vi "IV.vi"(2 "Run uninterrupted?":bool, 3 "Device Category IN:":string(combo)="Short Strip" caption="Device Category:", 4 "Batch No. IN:":string caption="Batch No.:", 5 "Sensor Serial No. IN:":string caption="Sensor Serial No.:", 6 "DB Serial No. IN:":string caption="DB Serial No.:") -> (0 "Done!":bool)   [LabVIEW 2018]
doc: "Performs IV measurements according to ATLAS ITk Quality Control Specifications."
uses:
  general_VIs/globals/QC_MeasurementSetup.vi
  general_VIs/globals/QC_RunInformation.vi
  InstrControl/InstrumentSetup.vi
  InstrControl/Switching/Switching.lvclass
  InstrControl/SupplyControl/SupplyControl.lvclass
  InstrControl/ArduinoControl/ArduinoControl.lvclass
  <vilib>/Analysis/NI_AALBase.lvlib
  InstrControl/InstrControl.lvclass
panel:
  out "Tab Control 2":enum32{"IV Setup", "IV Scan"}(tab)
  in  "V_breakdown limit [V]":dbl=-500.0
  in  "Set current limit?":bool
  in  "Current Limit [µA]":dbl=1000.0 min=0.0001 format="%.3f"
  in  "Measurement Configurations":bool
  in  "hold steps IN":i32=6 caption="hold steps"
  in  "Initial volts [V] IN":dbl caption="Initial volts [V]"
  in  "Final volts [V] IN":dbl=-700.0 caption="Final volts [V]"
  in  "step [V] IN":dbl=10.0 caption="step [V]" format="%.1f"
  in  "step interval [s] IN":i32=10 caption="step interval [s]"
  in  "Continue":bool
  in  "Quit":bool
  out "hold steps":i32
  out "RH":dbl[](array[numeric]) caption="RH [%]" format="%#.2f"
  out "Temp.":dbl[](array[numeric]) caption="Temp. [°C]" format="%#.2f"
  out "Current":dbl[](array[numeric]) caption="Current [nA]"
  out "Volts":dbl[](array[numeric]) caption="Volts [V]"
  out "step interval [s]":i32=10
  out "step [V]":dbl=10.0 format="%.1f"
  out "Final volts [V]":dbl=-700.0 format="%.1f"
  out "Initial volts [V]":dbl format="%.1f"
  out "Igraph":cluster{dbl[], dbl[]}(graph)
  in  "Scales":T1(ring)
  in  "Iscale":enum16{"nanoAmps", "microAmps", "milliAmps"}(ring)
  out "positive ramp?":bool
  out "Tab Control":enum32{"IV Setup", "IV Scan"}(tab)
  in  "Hardware Configurations":bool
  in  "User:":string(combo)="Christoph"
  in  "IV Supply":string(combo)="Keithley 2410"
  in  "Temperature":enum16{"Read Arduino", "Enter manually"}(ring)
  in  "Manufacturer:":string(combo)="Hamamatsu"
  in  "abort":bool
  out "Device Category:":string
  out "DB Serial No.:":string
  out "Current Volts:":dbl format="%.2f"
  in  "quit (no save)":bool
  in  "Quit & Save":bool
  out "Bias On/Off:":bool
  out "STATUS 1":string
  out "Initiated:":string
  out "Sensor No.:":string
  out "No of steps":u32
  out "Current reading No.":u32
  out "Last reading at:":string
  # "University of\nCambridge"
  # "Strip Sensor QC: IV"
  # "Vertical Scale:"
  # "Measurement Configuration"
  # "IV Scan parameters:"
  # "Last 5 readings:"
  # "n-4"
  # "n-3"
  # "n-2"
  # "n-1"
  # "n"
  # "DUT Description"
  # "Hardware"
  # "DUT & Test Description:"
  # "Current status:"
  # "Rdg No:"
  # "out of"
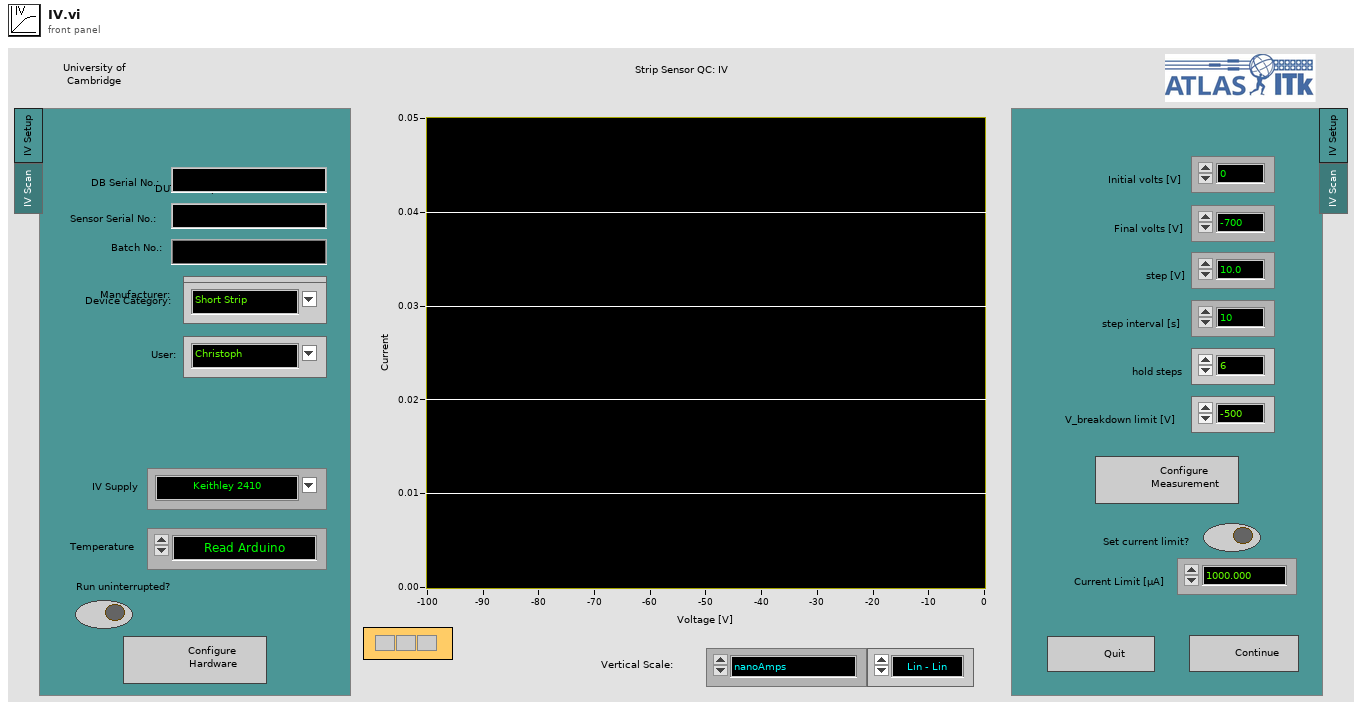
[diagram p1: front panel]
types:
  T1 = enum16{"Lin - Lin", "Log - Lin", "Lin - Log", "Log - log"}
  T2 = enum16{"Supply", "LCR", "Multimeter", "Switching"}
  T3 = enum16{"Reset", "Read Array", "Read Element", "Write Element", "Write Array", "Add Element", "Add Array"}
  T4 = enum16{"Reset", "Ground", "Striptest SMU", "Striptest LCR", "IV", "CV", "Interstrip Cap", "Interstrip Res"}
  T5 = enum32{"IV", "CV", "Stability", "Striptest", "Cis", "Ris", "PTP"}
  T6 = cluster{"Sensor Serial No.:":string, "Wafer Serial No.:":string, "Batch:":string, "Manufacturer:":string, "Device Category:":string, "Database Serial No.:":string, "Date Initiated:":string, "Time Initiated:":string, "Test":string, "Instruments used:":string, "Probeplan used:":string, "End of Run comment:":string, "User:":string}
  T7 = cluster{"Institute":string, "Manufacturers":string[], "Devices":string[], "Serialnumbers Lookup DB":string, "Data directory":string, "Backup & screenshot directory":string, "List of known users":string[]}
  T8 = cluster{"Supply":refnum<class "SupplyControl.lvclass">, "Initial Voltage [V]":dbl, "Final Voltage [V]":dbl, "Step Size [V]":dbl, "Step Interval [s]":i32, "Number Of Steps":u32, "Ramp down steps [V]":dbl, "Ramp down Interval [s]":i32, "hold steps":i32, "Set Current Limit?":bool, "Current Limit [µA]":dbl, "Temperature Readout":enum16{"Read Arduino", "Enter manually"}, "Arduino":refnum<class "ArduinoControl.lvclass">, "Supply Name":string, "V_breakdown Limit [V]":dbl, "Switching":refnum<class "Switching.lvclass">, "Matrix used?":bool, "Matrix X Channels":cluster{"Bias Supply / SMU LO":i32, "Bias Supply / SMU HI":i32, "CV Box LO":i32, "CV Box HI":i32, "CV Box LO IN":i32, "CV Box HI IN":i32, "Volt meter LO":i32, "Volt meter HI":i32, "Mux1 C1":i32, "Mux1 C2":i32, "Mux2 C1":i32, "Mux2 C2":i32}, "IV Test?":bool}
  T9 = cluster{"VISA address":refnum<visa-resource-name>, "T sensor":enum16{"SHT", "DS"}, "Arduino":refnum<class "ArduinoControl.lvclass">}
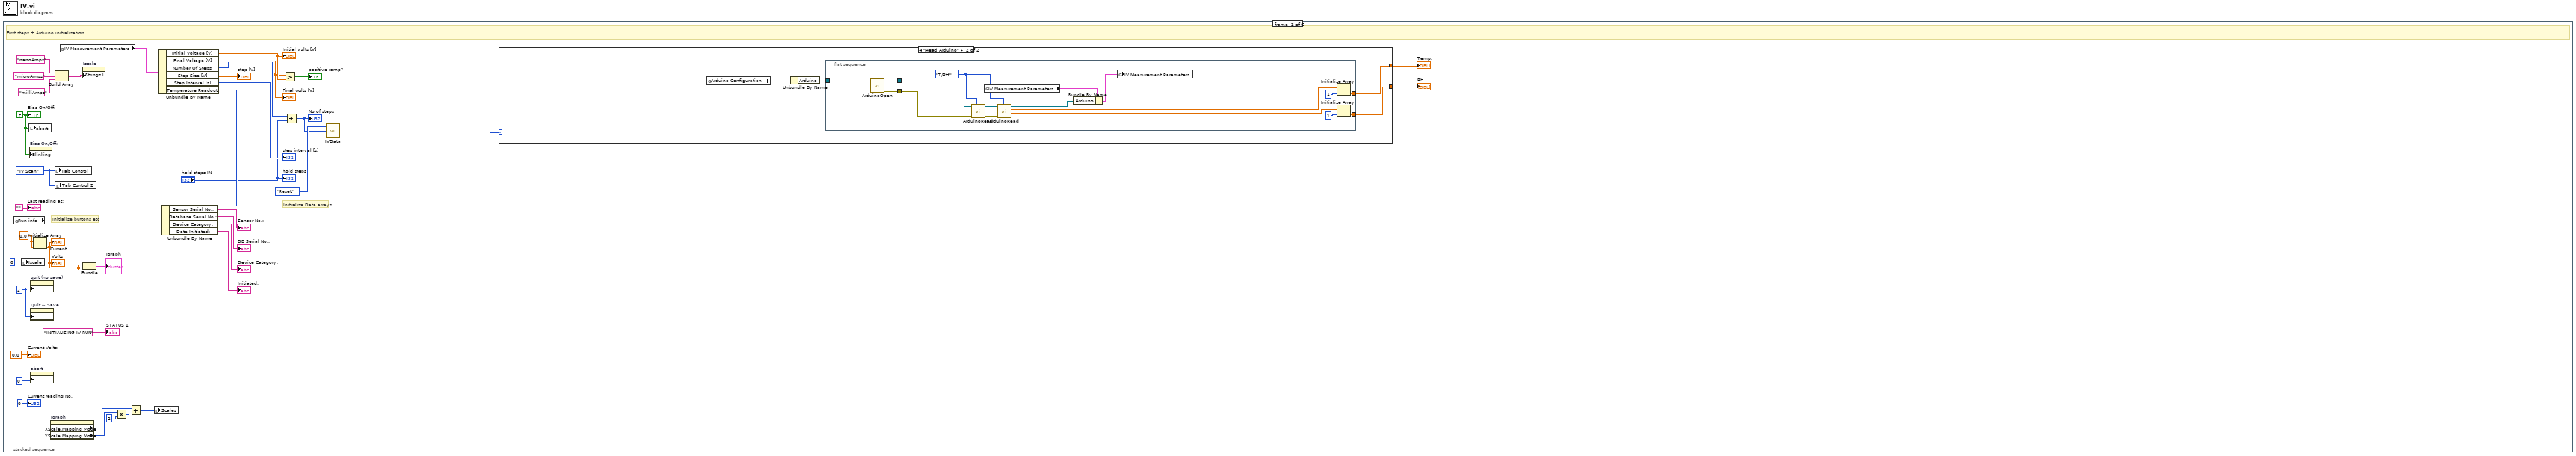
[diagram p0: block diagram]
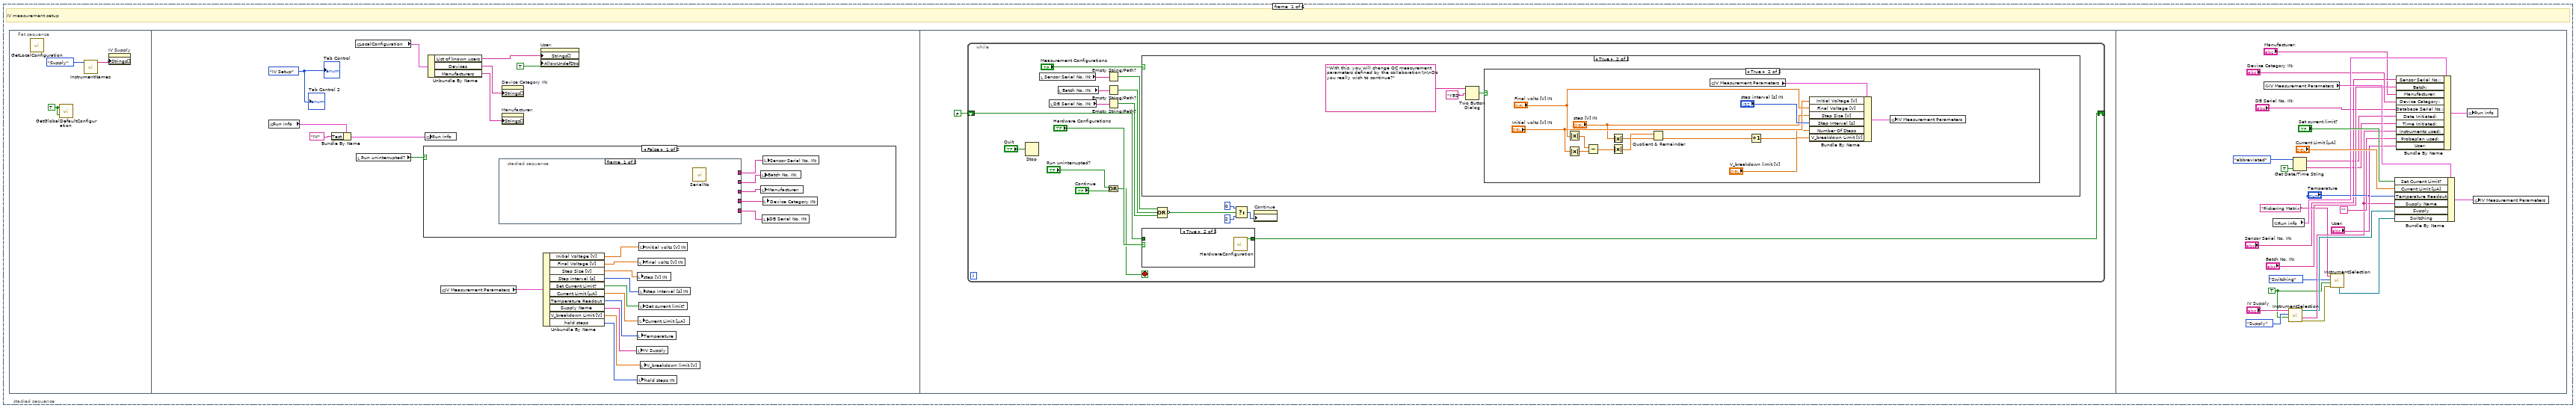
[diagram p2: hidden frame]
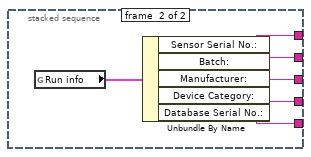
[diagram p3: hidden frame]
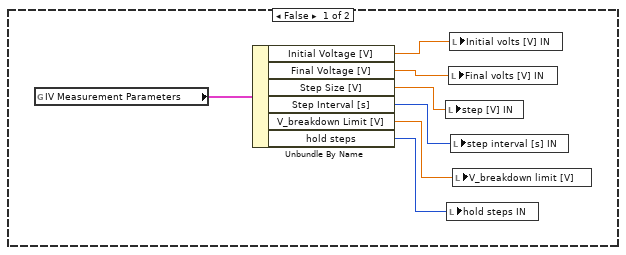
[diagram p6: hidden frame]
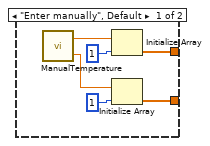
[diagram p8: hidden frame]
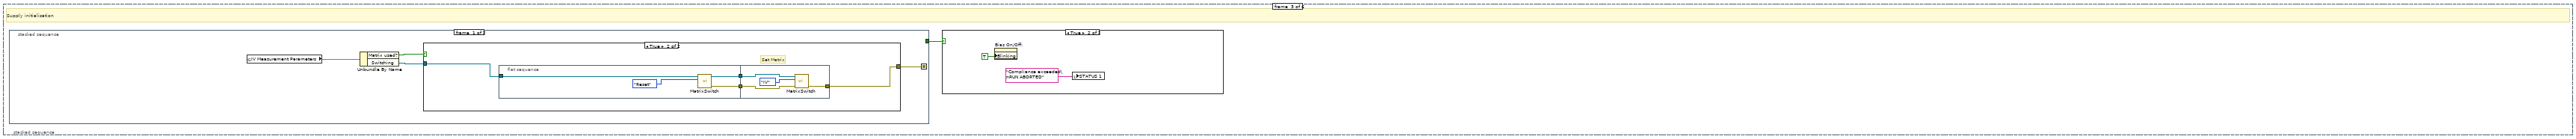
[diagram p9: hidden frame]
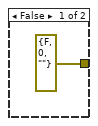
[diagram p10: hidden frame]
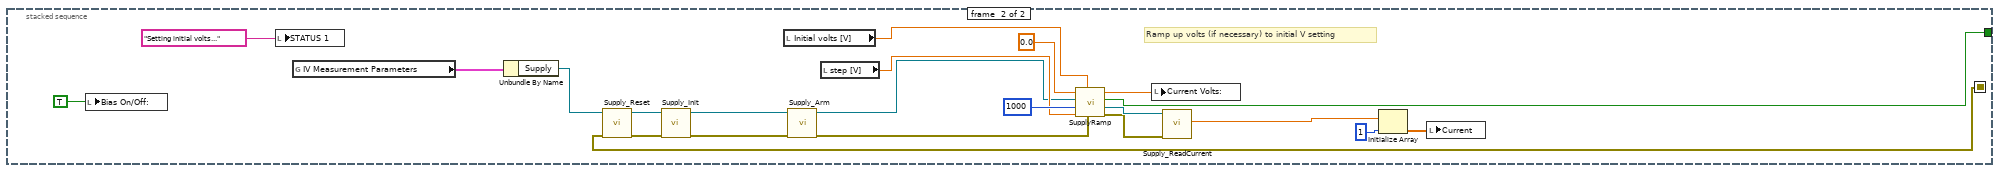
[diagram p11: hidden frame]
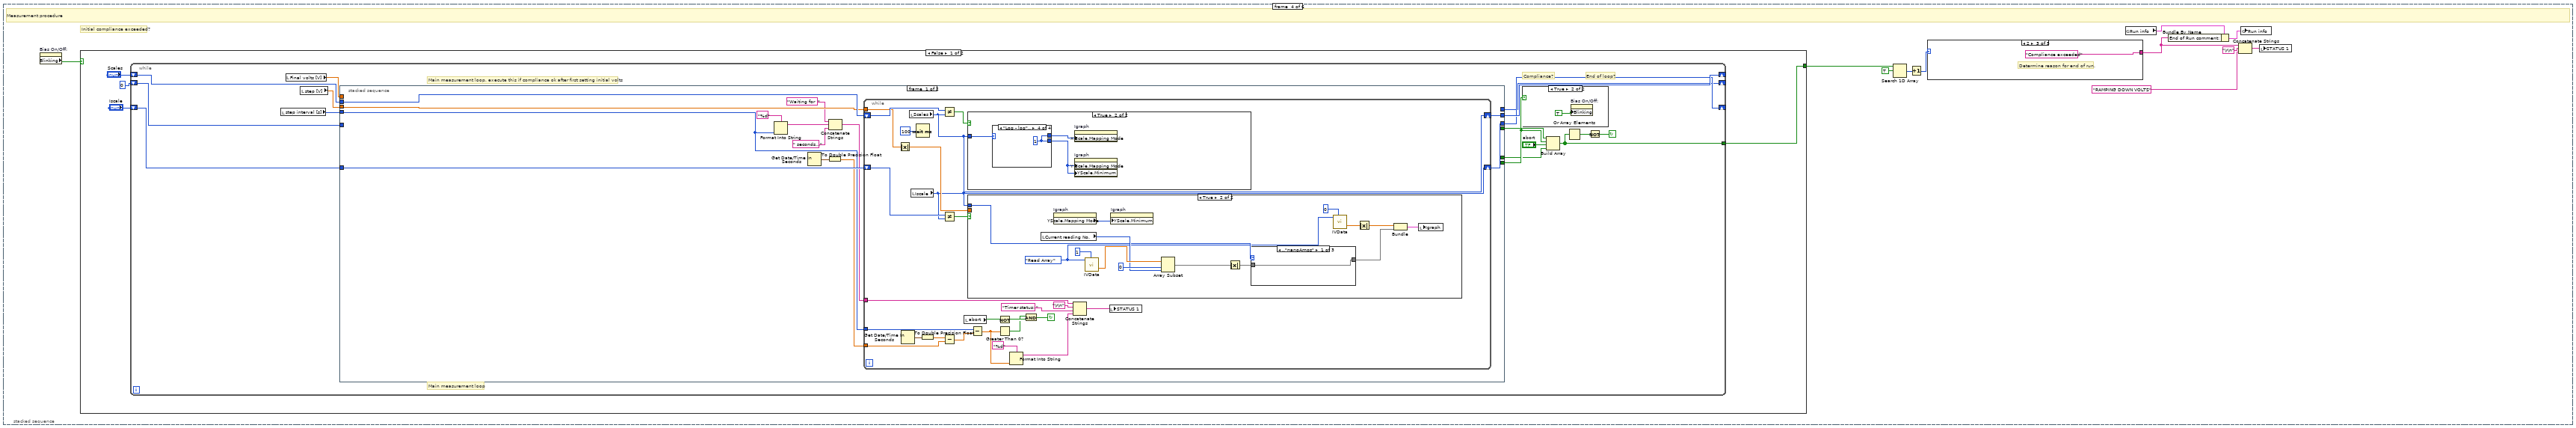
[diagram p13: hidden frame]
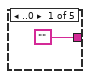
[diagram p14: hidden frame]
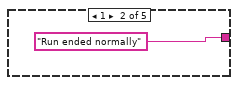
[diagram p15: hidden frame]
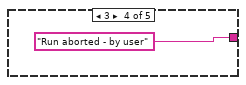
[diagram p16: hidden frame]
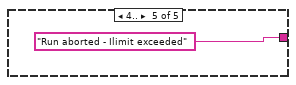
[diagram p17: hidden frame]
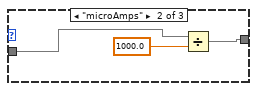
[diagram p19: hidden frame]
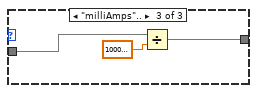
[diagram p20: hidden frame]
diagram:
  n1 = stacked-sequence {
    frame #0 {
      # "IV measurement setup"
      n2 = flat-sequence {
        frame #0 {
          w3 = TRUE
          n3 = call "GetLocalConfiguration.vi"() -> ()  [unwired: 3 in, 1 out]
          n4 = call "GetGlobalDefaultConfiguration.vi"("DO NOT override instruments"=w3, "Read defaults?"=w3) -> ()  [unwired: 1 in, 1 out]
          n5 = call "InstrumentNames.vi"("Instrument type"=T2."Supply") -> ("Instrument names"=w1:string[])  [unwired: 9 in, 1 out]
          n6 = property on="IV Supply" class="CmbBox"("Strings[]"=w1) -> ()  [unwired: 2 in, 2 out]
        }
        frame #1 {
          w12 = enum32{"IV Setup", "IV Scan"}."IV Setup" ("Tab Control")
          n7 = global read "QC_RunInformation.vi" "Run info"() -> (w15:T6)
          n8 = Bundle By Name(cluster=w15, "Test"="IV") -> (w13:T6)
          n9 = global read "QC_RunInformation.vi" "LocalConfiguration"() -> (w19:T7)
          n10 = local read "Run uninterrupted?"() -> (w16:bool)
          n11 = case shown="False" w16 {
            frame False {
              n12 = stacked-sequence {
                tunnel: [_ w35] -> w28
                tunnel: [_ w34] -> w27
                tunnel: [_ w33] -> w26
                tunnel: [_ w32] -> w29
                tunnel: [_ w30] -> w25
                frame #0 {
                  n13 = call "SerialNo.vi"() -> ()  [unwired: 5 in, 1 out]
                }
                frame #1 {
                  n14 = global read "QC_RunInformation.vi" "Run info"() -> (w31:T6)
                  n15 = Unbundle By Name(w31) -> ("Sensor Serial No.:"=w35:string, "Batch:"=w34:string, "Manufacturer:"=w33:string, "Device Category:"=w32:string, "Database Serial No.:"=w30:string)
                }
              }
              n16 = local write "Batch No. IN:"(w27) -> ()
              n17 = local write "Manufacturer:"(w26) -> ()
              n18 = local write "DB Serial No. IN:"(w25) -> ()
              n19 = local write "Device Category IN:"(w29) -> ()
              n20 = local write "Sensor Serial No. IN:"(w28) -> ()
            }
            frame True {
            }
          }
          n21 = global write "QC_RunInformation.vi" "Run info"(w13) -> ()
          n22 = Unbundle By Name(w19) -> ("List of known users"=w18:string[], "Devices"=w5:string[], "Manufacturers"=w4:string[])
          n23 = global read "QC_MeasurementSetup.vi" "IV Measurement Parameters"() -> (w22:T8)
          n24 = property on="Device Category IN:" class="CmbBox"("Strings[]"=w5) -> ()  [unwired: 2 in, 2 out]
          n25 = property on="Manufacturer:" class="CmbBox"("Strings[]"=w4) -> ()  [unwired: 2 in, 2 out]
          n26 = property on="User:" class="CmbBox"("Strings[]"=w18, "AllowUndefStrs"=TRUE) -> ()  [unwired: 2 in, 2 out]
          n27 = Unbundle By Name(w22) -> ("Initial Voltage [V]"=w10:dbl, "Final Voltage [V]"=w9:dbl, "Step Size [V]"=w8:dbl, "Step Interval [s]"=w11:i32, "Set Current Limit?"=w21:bool, "Current Limit [µA]"=w20:dbl, "Temperature Readout"=w24:enum16{"Read Arduino", "Enter manually"}, "Supply Name"=w23:string, "V_breakdown Limit [V]"=w7:dbl, "hold steps"=w6:i32)
          n28 = local write "IV Supply"(w23) -> ()
          n29 = local write "step [V] IN"(w8) -> ()
          n30 = local write "Temperature"(w24) -> ()
          n31 = local write "hold steps IN"(w6) -> ()
          n32 = local write "Final volts [V] IN"(w9) -> ()
          n33 = local write "Current Limit [µA]"(w20) -> ()
          n34 = local write "Initial volts [V] IN"(w10) -> ()
          n35 = local write "Set current limit?"(w21) -> ()
          n36 = local write "step interval [s] IN"(w11) -> ()
          n37 = local write "V_breakdown limit [V]"(w7) -> ()
          "Tab Control" <- w12
          "Tab Control 2" <- w12
        }
        frame #2 {
          n38 = while {
            shift-right: [w44] -> _
            shift-left: FALSE -> [w43]
            stop <- w40 stop-if-true
            n39 = Stop(stop? (T)="Quit") -> ()
            n40 = local read "Sensor Serial No. IN:"() -> (w53:string)
            n41 = local read "DB Serial No. IN:"() -> (w38:string)
            n42 = local read "Batch No. IN:"() -> (w46:string)
            n43 = Empty String/Path?(string/path=w53) -> (empty?=w52:bool)
            n44 = Empty String/Path?(string/path=w46) -> (empty?=w45:bool)
            n45 = Empty String/Path?(string/path=w38) -> (empty?=w37:bool)
            n46 = Or(x="Run uninterrupted?", y="Continue") -> (x .or. y?=w40:bool)
            n47 = case shown="True" "Measurement Configurations" {
              frame False {
              }
              frame True {
                n48 = Two Button Dialog(message="With this, you will change QC measurement parameters defined by the collaboration!\n\nDo you really wish to continue?", 2:"YES") -> (T button?=w55:bool)  [unwired: 1 in]
                n49 = case shown="True" w55 {
                  frame False {
                    n50 = global read "QC_MeasurementSetup.vi" "IV Measurement Parameters"() -> (w64:T8)
                    n51 = Unbundle By Name(w64) -> ("Initial Voltage [V]"=w62:dbl, "Final Voltage [V]"=w63:dbl, "Step Size [V]"=w61:dbl, "Step Interval [s]"=w60:i32, "V_breakdown Limit [V]"=w59:dbl, "hold steps"=w58:i32)
                    n52 = local write "step [V] IN"(w61) -> ()
                    n53 = local write "hold steps IN"(w58) -> ()
                    n54 = local write "Final volts [V] IN"(w63) -> ()
                    n55 = local write "Initial volts [V] IN"(w62) -> ()
                    n56 = local write "step interval [s] IN"(w60) -> ()
                    n57 = local write "V_breakdown limit [V]"(w59) -> ()
                  }
                  frame True {
                    n58 = Absolute Value(x="Final volts [V] IN") -> (abs(x)=w74:dbl)
                    n59 = Absolute Value(x="Initial volts [V] IN") -> (abs(x)=w73:dbl)
                    n60 = Subtract(x=w74, y=w73) -> (x-y=w68:dbl)
                    n61 = Absolute Value(x="step [V] IN") -> (abs(x)=w69:dbl)
                    n62 = Absolute Value(x=w68) -> (abs(x)=w70:dbl)
                    n63 = Quotient & Remainder(x=w70, y=w69) -> (floor(x/y)=w66:dbl)  [unwired: 1 out]
                    n64 = global read "QC_MeasurementSetup.vi" "IV Measurement Parameters"() -> (w78:T8)
                    n65 = Increment(x=w66) -> (x+1=w65:dbl)
                    n66 = Bundle By Name(cluster=w78, "Initial Voltage [V]"="Initial volts [V] IN", "Final Voltage [V]"="Final volts [V] IN", "Step Size [V]"="step [V] IN", "Step Interval [s]"="step interval [s] IN", "Number Of Steps"=w65, "V_breakdown Limit [V]"="V_breakdown limit [V]") -> (w75:T8)
                    n67 = global write "QC_MeasurementSetup.vi" "IV Measurement Parameters"(w75) -> ()
                  }
                }
              }
            }
            n68 = case shown="True" "Hardware Configurations" {
              tunnel: [w79 w80] -> w44
              tunnel: w43 -> [w79 _]
              frame False {
              }
              frame True {
                n69 = call "HardwareConfiguration.vi"() -> ("configured?"=w80:bool)  [unwired: 11 in]
              }
            }
            n70 = Compound Arithmetic op=OR(w52, w45, w37) -> (invert w51:bool)
            n71 = Select(t=0, s=w51, f=2) -> (s? t:f=w48:i32)
            n72 = property on="Continue" class="Bool"("DisabledEnum"=w48) -> ()  [unwired: 2 in, 2 out]
          }
        }
        frame #3 {
          w88 = TRUE
          n73 = global read "QC_MeasurementSetup.vi" "IV Measurement Parameters"() -> (w106:T8)
          n74 = global read "QC_RunInformation.vi" "Run info"() -> (w101:T6)
          n75 = call "InstrumentSelection.vi"("Verify GPIB address"=w88, "Instrument type"=T2."Supply", "Instrument name IN"="IV Supply") -> ("error out"=w90:errorcluster, "Instrument name OUT"=w93:string, "Supply"=w92:refnum<class "SupplyControl.lvclass">)  [unwired: 3 in, 3 out]
          n76 = Get Date/Time String(date format (0)=enum16{"short", "long", "abbreviated"}."abbreviated", want seconds? (F)=TRUE) -> (date string=w82:string, time string=w81:string)  [unwired: 1 in]
          n77 = call "InstrumentSelection.vi"("error in (no error)"=w90, "Verify GPIB address"=w88, "Instrument type"=T2."Switching", "Instrument name IN"="Pickering Matrix") -> ("Switching"=w89:refnum<class "Switching.lvclass">)  [unwired: 2 in, 5 out]
          n78 = Bundle By Name(cluster=w106, "Set Current Limit?"="Set current limit?", "Current Limit [µA]"="Current Limit [µA]", "Temperature Readout"="Temperature", "Supply Name"=w93, "Supply"=w92, "Switching"=w89) -> (w107:T8)
          n79 = Bundle By Name(cluster=w101, "Sensor Serial No.:"="Sensor Serial No. IN:", "Batch:"="Batch No. IN:", "Manufacturer:"="Manufacturer:", "Device Category:"="Device Category IN:", "Database Serial No.:"="DB Serial No. IN:", "Date Initiated:"=w82, "Time Initiated:"=w81, "Instruments used:"=w93, "Probeplan used:"="", "User:"="User:") -> (w100:T6)
          n80 = global write "QC_RunInformation.vi" "Run info"(w100) -> ()
          n81 = global write "QC_MeasurementSetup.vi" "IV Measurement Parameters"(w107) -> ()
        }
      }
    }
    frame #1 {
      w109 = enum32{"IV Setup", "IV Scan"}."IV Scan" ("Tab Control")
      w129 = 2
      w136 = 0.0
      w128 = FALSE ("Visible")
      # "Initialise buttons etc"
      # "Initialise Data arrays"
      # "First steps + Arduino initialisation"
      n82 = global read "QC_RunInformation.vi" "Run info"() -> (w145:T6)
      n83 = local write "Iscale"(u16 0 ("Scale")) -> ()
      n84 = local write "abort"(w128) -> ()
      n85 = property on="Bias On/Off:" class="Bool (strict)"("Blinking"=w128) -> ()  [unwired: 2 in, 2 out]
      n86 = property on="quit (no save)" class="Bool"("DisabledEnum"=w129) -> ()  [unwired: 2 in, 2 out]
      n87 = property on="Quit & Save" class="Bool"("DisabledEnum"=w129) -> ()  [unwired: 2 in, 2 out]
      n88 = property on="abort" class="Bool (strict)"("DisabledEnum"=0) -> ()  [unwired: 2 in, 2 out]
      n89 = Initialize Array(w136, w136) -> (w111:dbl[])
      "Volts" <- w111
      "Current" <- w111
      n90 = property on="Igraph" class="XYGraph (strict)"() -> ("XScale.Mapping Mode"=w121:u8, "YScale.Mapping Mode"=w120:u8)  [unwired: 2 in, 2 out]
      n91 = local write "Tab Control"(w109) -> ()
      n92 = Build Array("nanoAmps", "microAmps", "milliAmps") -> (w142:string[])
      n93 = local write "Tab Control 2"(w109) -> ()
      n94 = global read "QC_MeasurementSetup.vi" "IV Measurement Parameters"() -> (w117:T8)
      n95 = property on="Iscale" class="Enum (strict)"("Strings []"=w142) -> ()  [unwired: 2 in, 2 out]
      n96 = Bundle(w111, w111) -> (→"Igraph":cluster{dbl[], dbl[]})  [unwired: 1 in]
      n97 = Multiply(x=w120, y=2) -> (x*y=w123:i32)
      n98 = Add(x=w121, y=w123) -> (x+y=w119:i32)
      n99 = local write "Scales"(w119) -> ()
      n100 = Unbundle By Name(w117) -> ("Initial Voltage [V]"=w127:dbl, "Final Voltage [V]"=w126:dbl, "Number Of Steps"=w113:u32, "Step Size [V]"=→"step [V]":dbl, "Step Interval [s]"=→"step interval [s]":i32, "Temperature Readout"=w130:enum16{"Read Arduino", "Enter manually"})
      "Initial volts [V]" <- w127
      "Final volts [V]" <- w126
      n101 = Unbundle By Name(w145) -> ("Sensor Serial No.:"=→"Sensor No.:":string, "Database Serial No.:"=→"DB Serial No.:":string, "Device Category:"=→"Device Category:":string, "Date Initiated:"=→"Initiated:":string)
      n102 = Greater?(x=w126, y=w127) -> (0:→"positive ramp?":bool)
      n103 = Add(x=w113, y="hold steps IN") -> (x+y=w112:u32)
      "No of steps" <- w112
      n104 = call "IVData.vi"("Action"=T3."Reset", "Array Size / Index"=w112) -> ()  [unwired: 3 in, 2 out]
      n105 = case shown="\"Read Arduino\"" w130 {
        tunnel: [w151 w158] -> w133
        tunnel: [w148 w157] -> w118
        frame "Enter manually", Default {
          n106 = call "ManualTemperature.vi"() -> ("Humidity [%] out"=w147:dbl, "Temperature [°C] out"=w152:dbl)
          n107 = Initialize Array(w152, 1) -> (w151:dbl[])
          n108 = Initialize Array(w147, 1) -> (w148:dbl[])
        }
        frame "Read Arduino" {
          n109 = global read "InstrumentSetup.vi" "Arduino Configuration"() -> (w154:T9)
          n110 = Unbundle By Name(w154) -> ("Arduino"=w153:refnum<class "ArduinoControl.lvclass">)
          n111 = flat-sequence {
            tunnel: [w159] -> w156
            tunnel: [w161] -> w155
            tunnel: w153 -> [w160]
            tunnel: [w175] -> w158
            tunnel: [w172] -> w157
            tunnel: w156 -> [w166]
            tunnel: w155 -> [w165]
            frame #0 {
              n112 = call "ArduinoOpen.vi"("ArduinoControl in"=w160) -> ("error out"=w161:errorcluster, "ArduinoControl out"=w159:refnum<class "ArduinoControl.lvclass">)  [unwired: 9 in]
            }
            frame #1 {
              w162 = enum16{"T/RH", "Interlock", "Edgesense"}."T/RH" ("Arduino function")
              n113 = call "ArduinoRead.vi"("Arduino function"=w162, "error in (no error)"=w165, "ArduinoControl in"=w166) -> ("error out"=w164:errorcluster, "ArduinoControl out"=w163:refnum<class "ArduinoControl.lvclass">)  [unwired: 3 in, 4 out]
              n114 = global read "QC_MeasurementSetup.vi" "IV Measurement Parameters"() -> (w168:T8)
              n115 = call "ArduinoRead.vi"("Arduino function"=w162, "error in (no error)"=w164, "ArduinoControl in"=w163) -> ("rel. Humidity [%]"=w170:dbl, "Temperature [°C]"=w171:dbl, "ArduinoControl out"=w169:refnum<class "ArduinoControl.lvclass">)  [unwired: 3 in, 3 out]
              n116 = Bundle By Name(cluster=w168, "Arduino"=w169) -> (w167:T8)
              n117 = global write "QC_MeasurementSetup.vi" "IV Measurement Parameters"(w167) -> ()
              n118 = Initialize Array(w171, 1) -> (w175:dbl[])
              n119 = Initialize Array(w170, 1) -> (w172:dbl[])
            }
          }
        }
      }
      "Temp." <- w133
      "RH" <- w118
      "STATUS 1" <- "INITIALISING IV RUN"
      "Bias On/Off:" <- w128
      "Last reading at:" <- ""
      "Current reading No." <- u32 0 ("Current reading No.")
      "Current Volts:" <- 0.0 ("Current Volts:")
      "hold steps" <- "hold steps IN"
    }
    frame #2 {
      # "Supply initialisation"
      n120 = stacked-sequence {
        seq-local: [w178 _] -> [_ w194]
        tunnel: [_ w195] -> w176
        frame #0 {
          n121 = global read "QC_MeasurementSetup.vi" "IV Measurement Parameters"() -> (w177:T8)
          n122 = Unbundle By Name(w177) -> ("Matrix used?"=w180:bool, "Switching"=w179:refnum<class "Switching.lvclass">)
          n123 = case shown="True" w180 {
            tunnel: w179 -> [_ w182]
            tunnel: [errorcluster {"status"=FALSE, "code"=0, "source"=""} ("error constant") w183] -> w178
            frame False {
            }
            frame True {
              # "Set Matrix"
              n124 = flat-sequence {
                tunnel: [w189] -> w185
                tunnel: [w188] -> w184
                tunnel: w182 -> [w186]
                tunnel: w185 -> [w193]
                tunnel: w184 -> [w192]
                tunnel: [w191] -> w183
                frame #0 {
                  n125 = call-dynamic "MatrixSwitch.vi"("Action"=T4."Reset", "Switching in"=w186) -> ("error out"=w189:errorcluster, "Switching out"=w188:refnum<class "Switching.lvclass">)  [unwired: 7 in, 1 out]
                }
                frame #1 {
                  n126 = call-dynamic "MatrixSwitch.vi"("error in (no error)"=w193, "Action"=T4."IV", "Switching in"=w192) -> ("error out"=w191:errorcluster)  [unwired: 6 in, 2 out]
                }
              }
            }
          }
        }
        frame #1 {
          # "Ramp up volts (if necessary) to initial V setting"
          n127 = local write "Bias On/Off:"(TRUE ("Compliance?")) -> ()
          n128 = local write "STATUS 1"("Setting initial volts..." ("STATUS 1")) -> ()
          n129 = global read "QC_MeasurementSetup.vi" "IV Measurement Parameters"() -> (w211:T8)
          n130 = Unbundle By Name(w211) -> ("Supply"=w208:refnum<class "SupplyControl.lvclass">)
          n131 = call-dynamic "Supply_Reset.vi"("error in (no error)"=w194, "SupplyControl in"=w208) -> ("error out"=w213:errorcluster, "SupplyControl out"=w215:refnum<class "SupplyControl.lvclass">)  [unwired: 8 in]
          n132 = call-dynamic "Supply_Init.vi"("error in (no error)"=w213, "SupplyControl in"=w215) -> ("error out"=w212:errorcluster, "SupplyControl out"=w214:refnum<class "SupplyControl.lvclass">)  [unwired: 8 in]
          n133 = local read "Initial volts [V]"() -> (w203:dbl)
          n134 = call-dynamic "Supply_Arm.vi"("error in (no error)"=w212, "SupplyControl in"=w214) -> ("error out"=w201:errorcluster, "SupplyControl out"=w202:refnum<class "SupplyControl.lvclass">)  [unwired: 8 in]
          n135 = local read "step [V]"() -> (w204:dbl)
          n136 = call "SupplyRamp.vi"("error in"=w201, "Requested Voltage"=w203, "Step Size"=w204, "Step Delay"=1000, "Supply IN"=w202, "Starting Voltage"=0.0) -> ("error out"=w196:errorcluster, "Supply OUT"=w197:refnum<class "SupplyControl.lvclass">, "Compliance exceeded"=w195:bool, "Current Voltage"=w207:dbl)  [unwired: 2 in]
          n137 = local write "Current Volts:"(w207) -> ()
          n138 = call-dynamic "Supply_ReadCurrent.vi"("error in (no error)"=w196, "SupplyControl in"=w197) -> ("Current in nA"=w199:dbl)  [unwired: 7 in, 2 out]
          n139 = Initialize Array(w199, 1) -> (w198:dbl[])
          n140 = local write "Current"(w198) -> ()
        }
      }
      n141 = case shown="True" w176 {
        frame False {
        }
        frame True {
          n142 = property on="Bias On/Off:" class="Bool (strict)"("Blinking"=TRUE) -> ()  [unwired: 2 in, 2 out]
          n143 = local write "STATUS 1"("Compliance exceeded\nRUN ABORTED") -> ()
        }
      }
    }
    frame #3 {
      # "Initial compliance exceeded?"
      # "Measurement procedure"
      n144 = property on="Bias On/Off:" class="Bool (strict)"() -> ("Blinking"=w228:bool)  [unwired: 2 in, 2 out]
      n145 = case shown="False" w228 {
        tunnel: [w237 w487] -> w227
        frame False {
          n146 = while {
            shift-left: "Iscale" -> [w249]
            shift-right: [w248] -> _
            shift-left: "Scales" -> [w250]
            shift-right: [w251] -> _
            tunnel: [w247] -> w237
            shift-right: [w239] -> _
            shift-left: 0 -> [w240]
            stop <- w252 continue-if-true
            # "Main measurement loop"
            # "End of loop?"
            # "Compliance?"
            # "Main measurement loop. execute this if compliance ok after first setting initial volts"
            n147 = local read "step interval [s]"() -> (w244:i32)
            n148 = local read "Final volts [V]"() -> (w245:dbl)
            n149 = local read "step [V]"() -> (w246:dbl)
            n150 = stacked-sequence {
              tunnel: [w266 _] -> w251
              tunnel: w246 -> [w263 w330]
              tunnel: [_ w329] -> w242
              tunnel: w245 -> [_ w328]
              tunnel: w244 -> [w254 w327]
              tunnel: [_ w326] -> w243
              tunnel: w250 -> [w265 _]
              tunnel: w249 -> [w264 _]
              tunnel: [w262 _] -> w248
              tunnel: [_ w324] -> w238
              tunnel: w240 -> [_ w323]
              tunnel: [_ w322] -> w239
              frame #0 {
                n151 = Format Into String(format string="%d", w254) -> (resulting string=w259:string)  [unwired: 2 in, 1 out]
                n152 = Get Date/Time In Seconds() -> (seconds since 1Jan1904=w256:timestamp)
                n153 = To Double Precision Float(number=w256) -> (double precision float=w257:dbl)
                n154 = Concatenate Strings("Waiting for  ", w259, " seconds...") -> (w255:string)
                n155 = while {
                  tunnel: w263 -> [w275]
                  shift-left: w264 -> [w279]
                  shift-right: [w272] -> w262
                  shift-left: w265 -> [w280]
                  shift-right: [w281] -> w266
                  tunnel: w255 -> [w273]
                  tunnel: w254 -> [w285]
                  tunnel: w257 -> [w286]
                  stop <- w287 continue-if-true
                  n156 = Absolute Value(x=w275) -> (abs(x)=w274:dbl)
                  n157 = Get Date/Time In Seconds() -> (seconds since 1Jan1904=w271:timestamp)
                  n158 = local read "Scales"() -> (w281:T1)
                  n159 = local read "Iscale"() -> (w272:enum16{"nanoAmps", "microAmps", "milliAmps"})
                  n160 = Wait (ms)(milliseconds to wait=u32 100) -> ()  [unwired: 1 out]
                  n161 = To Double Precision Float(number=w271) -> (double precision float=w291:dbl)
                  n162 = Not Equal?(x=w280, y=w281) -> (x != y?=w282:bool)
                  n163 = Not Equal?(x=w279, y=w272) -> (x != y?=w270:bool)
                  n164 = Subtract(x=w291, y=w286) -> (x-y=w268:dbl)
                  n165 = local read "abort"() -> (w284:bool)
                  n166 = case shown="True" w282 {
                    tunnel: w281 -> [_ w315]
                    frame False {
                    }
                    frame True {
                      n167 = case shown="\"Log - log\".." w315 {
                        tunnel: [w316 1 0 w321] -> w314
                        tunnel: [w316 0 1 w321] -> w313
                        frame .."Lin - Lin" {
                          w316 = 0
                        }
                        frame "Log - Lin" {
                        }
                        frame "Lin - Log" {
                        }
                        frame "Log - log".. {
                          w321 = 1
                        }
                      }
                      n168 = property on="Igraph" class="XYGraph (strict)"("X Scale.Mapping Mode"=w314) -> ()  [unwired: 2 in, 2 out]
                      n169 = property on="Igraph" class="XYGraph (strict)"("Y Scale.Mapping Mode"=w313, "YScale.Minimum"=w313) -> ()  [unwired: 2 in, 2 out]
                    }
                  }
                  n170 = case shown="True" w270 {
                    tunnel: w274 -> [_ _]
                    tunnel: w272 -> [_ w300]
                    frame False {
                    }
                    frame True {
                      w294 = T3."Read Array" ("Action")
                      n171 = local read "Current reading No."() -> (w302:u32)
                      n172 = property on="Igraph" class="XYGraph (strict)"() -> ("YScale.Mapping Mode"=w296:u8)  [unwired: 2 in, 2 out]
                      n173 = call "IVData.vi"("Action"=w294, "Array No."=u32 1 ("Action")) -> ("Array OUT"=w303:dbl[])  [unwired: 3 in, 1 out]
                      n174 = property on="Igraph" class="XYGraph (strict)"("YScale.Minimum"=w296) -> ()  [unwired: 2 in, 2 out]
                      n175 = Array Subset(array=w303, index=0, length=w302) -> (w299:dbl[])
                      n176 = Absolute Value(x=w299) -> (abs(x)=w298:dbl[])
                      n177 = case shown="..\"nanoAmps\"" w300 {
                        tunnel: [w306 w307 w311] -> w305
                        tunnel: w298 -> [w306 w309 w312]
                        frame .."nanoAmps" {
                        }
                        frame "microAmps" {
                          n178 = Divide(x=w309, y=1000.0) -> (x/y=w307:dbl[])
                        }
                        frame "milliAmps".. {
                          n179 = Divide(x=w312, y=1000000.0) -> (x/y=w311:dbl[])
                        }
                      }
                      n180 = call "IVData.vi"("Action"=w294, "Array No."=u32 0 ("Action")) -> ("Array OUT"=w293:dbl[])  [unwired: 3 in, 1 out]
                      n181 = Absolute Value(x=w293) -> (abs(x)=w292:dbl[])
                      n182 = Bundle(w292, w305) -> (w301:cluster{dbl[], dbl[]})  [unwired: 1 in]
                      n183 = local write "Igraph"(w301) -> ()
                    }
                  }
                  n184 = Subtract(x=w285, y=w268) -> (x-y=w267:dbl)
                  n185 = Not(x=w284) -> (.not. x?=w290:bool)
                  n186 = Greater Than 0?(x=w267) -> (x > 0?=w269:bool)
                  n187 = Format Into String(format string="%d", w267) -> (resulting string=w289:string)  [unwired: 2 in, 1 out]
                  n188 = And(x=w269, y=w290) -> (x .and. y?=w287:bool)
                  n189 = Concatenate Strings(w273, "\r\n", "Timer status: ", w289) -> (w283:string)
                  n190 = local write "STATUS 1"(w283) -> ()
                }
              }
              frame #1 {
                n191 = local read "abort"() -> (w325:bool)
                n192 = case shown="False" w325 {
                  tunnel: [w338 w484] -> w326
                  tunnel: w327 -> [w337 _]
                  tunnel: w328 -> [w336 _]
                  tunnel: [w334 w484] -> w329
                  tunnel: w330 -> [w335 _]
                  tunnel: [w333 w484] -> w324
                  tunnel: w323 -> [w332 w483]
                  tunnel: [w331 w483] -> w322
                  frame False {
                    n193 = stacked-sequence {
                      seq-local: [w353 _ _] -> [_ w388 _]
                      seq-local: [w348 _ _] -> [_ _ w448]
                      seq-local: [w347 _ _] -> [_ _ w449]
                      tunnel: w335 -> [_ w385 w454]
                      tunnel: w336 -> [_ _ w446]
                      tunnel: [_ _ w452] -> w338
                      tunnel: [_ _ w451] -> w334
                      tunnel: w337 -> [_ _ _]
                      tunnel: [w357 _ _] -> w333
                      tunnel: w332 -> [_ w386 w440]
                      tunnel: [_ _ w439] -> w331
                      frame #0 {
                        w351 = T3."Write Element" ("Action")
                        # "SMU data"
                        n194 = Get Date/Time String(want seconds? (F)=TRUE) -> (time string=w354:string)  [unwired: 2 in, 1 out]
                        n195 = local write "Last reading at:"(w354) -> ()
                        n196 = local write "STATUS 1"("Reading current ..." ("status")) -> ()
                        n197 = global read "QC_MeasurementSetup.vi" "IV Measurement Parameters"() -> (w346:T8)
                        n198 = Unbundle By Name(w346) -> ("Supply"=w340:refnum<class "SupplyControl.lvclass">, "Set Current Limit?"=w345:bool, "Current Limit [µA]"=w342:dbl, "Temperature Readout"=w344:enum16{"Read Arduino", "Enter manually"}, "Arduino"=w339:refnum<class "ArduinoControl.lvclass">)
                        n199 = local read "Current reading No."() -> (w350:u32)
                        n200 = case shown="\"Read Arduino\"" w344 {
                          tunnel: [w367 w373] -> w355
                          tunnel: [w364 w372] -> w349
                          tunnel: w339 -> [_ w371]
                          frame "Enter manually", Default {
                            n201 = local read "Temp."() -> (w369:dbl[])
                            n202 = local read "RH"() -> (w365:dbl[])
                            n203 = Index Array(array=w369, index=0) -> (element=w367:dbl)
                            n204 = Index Array(array=w365, index=0) -> (element=w364:dbl)
                          }
                          frame "Read Arduino" {
                            n205 = call "ArduinoRead.vi"("Arduino function"=enum16{"T/RH", "Interlock", "Edgesense"}."T/RH", "ArduinoControl in"=w371) -> ("rel. Humidity [%]"=w372:dbl, "Temperature [°C]"=w373:dbl)  [unwired: 4 in, 4 out]
                          }
                        }
                        n206 = local read "Current Volts:"() -> (w359:dbl)
                        n207 = Multiply(x=w342, y=1000.0) -> (x*y=w341:dbl)
                        n208 = call-dynamic "Supply_ReadCurrent.vi"("SupplyControl in"=w340) -> ("error out"=w347:errorcluster, "Current in nA"=w358:dbl, "SupplyControl out"=w348:refnum<class "SupplyControl.lvclass">)  [unwired: 8 in]
                        n209 = case shown="True" w345 {
                          tunnel: w358 -> [_ w378]
                          tunnel: w341 -> [_ w376]
                          tunnel: [FALSE w375] -> w357
                          frame False {
                          }
                          frame True {
                            n210 = Absolute Value(x=w378) -> (abs(x)=w377:dbl)
                            n211 = Greater?(x=w377, y=w376) -> (0:w375:bool)
                          }
                        }
                        n212 = Increment(x=w350) -> (x+1=w353:u32)
                        n213 = call "IVData.vi"("Action"=w351, "Array No."=u32 1, "Array Size / Index"=w350, "Data IN"=w358) -> ()  [unwired: 1 in, 2 out]
                        n214 = call "IVData.vi"("Action"=w351, "Array No."=0, "Array Size / Index"=w350, "Data IN"=w359) -> ()  [unwired: 1 in, 2 out]
                        n215 = local write "Current reading No."(w353) -> ()
                        n216 = call "IVData.vi"("Action"=w351, "Array No."=u32 2, "Array Size / Index"=w350, "Data IN"=w355) -> ()  [unwired: 1 in, 2 out]
                        n217 = call "IVData.vi"("Action"=w351, "Array No."=u32 3, "Array Size / Index"=w350, "Data IN"=w349) -> ()  [unwired: 1 in, 2 out]
                      }
                      frame #1 {
                        w381 = T3."Read Array" ("Action")
                        w398 = u32 5 ("y")
                        # "Update plots"
                        n218 = Greater Than 0?(x=w386) -> (x > 0?=w387:bool)
                        n219 = property on="Igraph" class="XYGraph (strict)"() -> ("YScale.Mapping Mode"=w389:u8)  [unwired: 2 in, 2 out]
                        n220 = Select(t=0.01, s=w387, f=w385) -> (s? t:f=w384:dbl)
                        n221 = property on="Igraph" class="XYGraph (strict)"("YScale.Minimum"=w389) -> ()  [unwired: 2 in, 2 out]
                        n222 = call "IVData.vi"("Action"=w381, "Array No."=1) -> ("Array OUT"=w400:dbl[])  [unwired: 3 in, 1 out]
                        n223 = Absolute Value(x=w384) -> ()  [unwired: 1 out]
                        n224 = Greater?(x=w388, y=w398) -> (0:w397:bool)
                        n225 = case shown="False" w397 {
                          tunnel: w388 -> [w404 w407]
                          tunnel: w398 -> [_ w406]
                          tunnel: [w404 w406] -> w396
                          tunnel: [0 w405] -> w394
                          frame False {
                          }
                          frame True {
                            n226 = Subtract(x=w407, y=w406) -> (x-y=w405:u32)
                          }
                        }
                        n227 = Array Subset(array=w400, index=0, length=w388) -> (w393:dbl[])
                        n228 = local read "Iscale"() -> (w399:enum16{"nanoAmps", "microAmps", "milliAmps"})
                        n229 = Absolute Value(x=w393) -> (abs(x)=w392:dbl[])
                        n230 = case shown="\"microAmps\"" w399 {
                          tunnel: [w432 w433 w436] -> w402
                          tunnel: w392 -> [w432 w435 w438]
                          frame .."nanoAmps" {
                          }
                          frame "microAmps" {
                            n231 = Divide(x=w435, y=1000.0) -> (x/y=w433:dbl[])
                          }
                          frame "milliAmps".. {
                            n232 = Divide(x=w438, y=1000000.0) -> (x/y=w436:dbl[])
                          }
                        }
                        n233 = call "IVData.vi"("Action"=w381, "Array No."=0) -> ("Array OUT"=w380:dbl[])  [unwired: 3 in, 1 out]
                        n234 = Absolute Value(x=w380) -> (abs(x)=w379:dbl[])
                        n235 = for {
                          N: 4 -> [_]
                          tunnel: w396 -> [w412]
                          tunnel: w394 -> [w411]
                          tunnel: w388 -> [w408]
                          i -> [w413]
                          n236 = call "IVData.vi"("Action"=T3."Read Array", "Array No."=w413) -> ("Array OUT"=w410:dbl[])  [unwired: 3 in, 1 out]
                          n237 = case shown="3.." w413 {
                            tunnel: w412 -> [w416 w420 _ _]
                            tunnel: w411 -> [w417 w421 _ _]
                            tunnel: w410 -> [w415 w419 w425 w430]
                            tunnel: w408 -> [_ _ w423 w428]
                            frame ..0 {
                              n238 = Array Subset(array=w415, index=w417, length=w416) -> (w414:dbl[])
                              n239 = local write "Volts"(w414) -> ()
                            }
                            frame 1 {
                              n240 = Array Subset(array=w419, index=w421, length=w420) -> (w418:dbl[])
                              n241 = local write "Current"(w418) -> ()
                            }
                            frame 2 {
                              n242 = Decrement(x=w423) -> (x-1=w422:u32)
                              n243 = Array Subset(array=w425, index=w422, length=1) -> (w424:dbl[])
                              n244 = local write "Temp."(w424) -> ()
                            }
                            frame 3.. {
                              n245 = Decrement(x=w428) -> (x-1=w427:u32)
                              n246 = Array Subset(array=w430, index=w427, length=1) -> (w429:dbl[])
                              n247 = local write "RH"(w429) -> ()
                            }
                          }
                        }
                        n248 = Bundle(w379, w402) -> (w390:cluster{dbl[], dbl[]})  [unwired: 1 in]
                        n249 = local write "Igraph"(w390) -> ()
                      }
                      frame #2 {
                        # "Increment volts and check for end of loop"
                        n250 = local read "positive ramp?"() -> (w450:bool)
                        n251 = local read "Current Volts:"() -> (w441:dbl)
                        n252 = case shown="False" w450 {
                          tunnel: w446 -> [w457 w461]
                          tunnel: w454 -> [w458 w464]
                          tunnel: [w456 w463] -> w442
                          tunnel: [w455 w460] -> w453
                          tunnel: w441 -> [w459 w462]
                          frame False {
                            n253 = Subtract(x=w459, y=w458) -> (x-y=w455:dbl)
                            n254 = Greater Or Equal?(x=w455, y=w457) -> (x >= y?=w456:bool)
                          }
                          frame True {
                            n255 = Add(x=w462, y=w464) -> (x+y=w460:dbl)
                            n256 = Less Or Equal?(x=w460, y=w461) -> (x <= y?=w463:bool)
                          }
                        }
                        n257 = Quotient & Remainder(x=w441, y=w446) -> (x-y*floor(x/y)=w447:dbl, floor(x/y)=w445:dbl)
                        n258 = Not Equal To 0?(x=w447) -> (x != 0?=w443:bool)
                        n259 = Equal To 0?(x=w445) -> (x = 0?=w444:bool)
                        n260 = Or(x=w443, y=w444) -> ()  [unwired: 1 out]
                        n261 = case shown="True" w442 {
                          tunnel: w453 -> [_ w479]
                          tunnel: [w468 FALSE] -> w452
                          tunnel: [FALSE w480] -> w451
                          tunnel: w441 -> [_ w477]
                          tunnel: w449 -> [_ w476]
                          tunnel: w448 -> [_ w475]
                          tunnel: w440 -> [w467 _]
                          tunnel: [w466 0] -> w439
                          frame False {
                            (unwired) TRUE
                            n262 = Increment(x=w467) -> (x+1=w466:i32)
                            n263 = local read "hold steps"() -> (w465:i32)
                            n264 = Greater Or Equal?(x=w467, y=w465) -> (x >= y?=w468:bool)
                          }
                          frame True {
                            n265 = local read "step [V]"() -> (w473:dbl)
                            n266 = call "SupplyRamp.vi"("error in"=w476, "Requested Voltage"=w479, "Step Size"=w473, "Step Delay"=100, "Supply IN"=w475, "Starting Voltage"=w477) -> ("error out"=w471:errorcluster, "Compliance exceeded"=w480:bool, "Current Voltage"=w474:dbl)  [unwired: 2 in, 1 out]
                            n267 = case shown="No Error" w471 {
                              tunnel: w474 -> [w482 _]
                              frame No Error {
                                n268 = local write "Current Volts:"(w482) -> ()
                              }
                              frame Error {
                              }
                            }
                            n269 = local write "STATUS 1"("Incrementing volts.") -> ()
                            n270 = property on="Bias On/Off:" class="Bool (strict)"("Blinking"=w480) -> ()  [unwired: 2 in, 2 out]
                          }
                        }
                      }
                    }
                  }
                  frame True {
                    w484 = FALSE
                  }
                }
              }
            }
            n271 = case shown="True" w242 {
              frame False {
              }
              frame True {
                n272 = property on="Bias On/Off:" class="Bool (strict)"("Blinking"=TRUE) -> ()  [unwired: 2 in, 2 out]
              }
            }
            n273 = Build Array(w243, w242, "abort", w238) -> (w247:bool[])
            n274 = Or Array Elements(Boolean array=w247) -> (logical OR=w253:bool)
            n275 = Not(x=w253) -> (.not. x?=w252:bool)
          }
        }
        frame True {
          w486 = FALSE
          # "compliance was exceeded when first voltage applied."
          # "Flag compliance as reason for end of run"
          n276 = local write "STATUS 1"("Run aborted - compliance exceeded.") -> ()
          n277 = Build Array(w486, TRUE, w486, w486) -> (w487:bool[])
        }
      }
      n278 = Search 1D Array(1D array=w227, element=TRUE) -> (index of element=w225:i32)  [unwired: 1 in]
      n279 = Increment(x=w225) -> (x+1=w224:i32)
      n280 = case shown="2" w224 {
        tunnel: ["" "Run ended normally" "Compliance exceeded" "Run aborted - by user" "Run aborted - Ilimit exceeded"] -> w219
        frame ..0 {
        }
        frame 1 {
        }
        frame 2 {
          # "Determine reason for end of run."
        }
        frame 3 {
        }
        frame 4.. {
        }
      }
      n281 = global read "QC_RunInformation.vi" "Run info"() -> (w223:T6)
      n282 = Bundle By Name(cluster=w223, "End of Run comment:"=w219) -> (w218:T6)
      n283 = Concatenate Strings(w219, "\r\n", "RAMPING DOWN VOLTS") -> (w222:string)
      n284 = global write "QC_RunInformation.vi" "Run info"(w218) -> ()
      n285 = local write "STATUS 1"(w222) -> ()
    }
    frame #4 {
      # "Ramp down and switch off supply"
      n286 = stacked-sequence {
        frame #0 {
          # "Tie up loose ends. Set volts to zero and switch to standby"
          # "Ramp down volts now"
          n287 = global read "QC_MeasurementSetup.vi" "IV Measurement Parameters"() -> (w498:T8)
          n288 = Unbundle By Name(w498) -> ("Supply"=w495:refnum<class "SupplyControl.lvclass">, "Ramp down steps [V]"=w497:dbl, "Ramp down Interval [s]"=w496:i32, "Switching"=w490:refnum<class "Switching.lvclass">, "Matrix used?"=w491:bool)
          n289 = Multiply(x=w496, y=1000) -> (x*y=w500:i32)
          n290 = local read "Current Volts:"() -> (w503:dbl)
          n291 = call "SupplyRamp.vi"("Requested Voltage"=0.0, "Step Size"=w497, "Step Delay"=w500, "Supply IN"=w495, "Starting Voltage"=w503) -> ("error out"=w494:errorcluster, "Supply OUT"=w493:refnum<class "SupplyControl.lvclass">, "Current Voltage"=w501:dbl)  [unwired: 3 in, 1 out]
          n292 = local write "Current Volts:"(w501) -> ()
          n293 = call-dynamic "Supply_Stby.vi"("error in (no error)"=w494, "SupplyControl in"=w493) -> ("error out"=w492:errorcluster)  [unwired: 8 in, 1 out]
          n294 = case shown="True" w491 {
            tunnel: w490 -> [_ w506]
            tunnel: w492 -> [_ w505]
            frame False {
            }
            frame True {
              n295 = call-dynamic "MatrixSwitch.vi"("error in (no error)"=w505, "Action"=T4."Reset", "Switching in"=w506) -> ()  [unwired: 6 in, 3 out]
            }
          }
        }
        frame #1 {
          w511 = 0
          n296 = local write "Bias On/Off:"(FALSE ("Visible")) -> ()
          n297 = local write "Current Volts:"(0.0 ("Current Volts:")) -> ()
          n298 = property on="Quit & Save" class="Bool"("DisabledEnum"=w511) -> ()  [unwired: 2 in, 2 out]
          n299 = property on="quit (no save)" class="Bool"("DisabledEnum"=w511) -> ()  [unwired: 2 in, 2 out]
          n300 = property on="abort" class="Bool (strict)"("DisabledEnum"=2) -> ()  [unwired: 2 in, 2 out]
          n301 = local write "STATUS 1"("Run finished. \nSave data?" ("STATUS 1")) -> ()
        }
        frame #2 {
          n302 = Current VI's Path() -> (path=w513:path)
          n303 = call "SaveJPEG.vi"("Test"="IV", "File Path Control"=w513) -> ()  [unwired: 1 in, 2 out]
        }
      }
    }
    frame #5 {
      # "Loop and await decision on whether to save or junk data"
      # "Display and save data"
      n304 = local read "Scales"() -> (w524:T1)
      n305 = local read "Iscale"() -> (w523:enum16{"nanoAmps", "microAmps", "milliAmps"})
      n306 = while {
        shift-left: w523 -> [w572]
        shift-right: [w571] -> _
        shift-left: w524 -> [w574]
        shift-right: [w573] -> _
        tunnel: ["Quit & Save"] -> w526
        tunnel: ["quit (no save)"] -> w525
        stop <- w569 continue-if-true
        n307 = local read "Scales"() -> (w573:T1)
        n308 = local read "Iscale"() -> (w571:enum16{"nanoAmps", "microAmps", "milliAmps"})
        n309 = Not Equal?(x=w574, y=w573) -> (x != y?=w567:bool)
        n310 = Not Equal?(x=w572, y=w571) -> (x != y?=w566:bool)
        n311 = case shown="True" w567 {
          tunnel: w573 -> [_ w601]
          frame False {
          }
          frame True {
            n312 = case shown="..\"Lin - Lin\"" w601 {
              tunnel: [w602 1 0 w607] -> w600
              tunnel: [w602 0 1 w607] -> w599
              frame .."Lin - Lin" {
                w602 = 0
              }
              frame "Log - Lin" {
              }
              frame "Lin - Log" {
              }
              frame "Log - log".. {
                w607 = 1
              }
            }
            n313 = property on="Igraph" class="XYGraph (strict)"("X Scale.Mapping Mode"=w600) -> ()  [unwired: 2 in, 2 out]
            n314 = property on="Igraph" class="XYGraph (strict)"("Y Scale.Mapping Mode"=w599, "YScale.Minimum"=w599) -> ()  [unwired: 2 in, 2 out]
          }
        }
        n315 = case shown="True" w566 {
          tunnel: w571 -> [_ w587]
          frame False {
          }
          frame True {
            w580 = T3."Read Array" ("Action")
            n316 = property on="Igraph" class="XYGraph (strict)"() -> ("YScale.Mapping Mode"=w583:u8)  [unwired: 2 in, 2 out]
            n317 = property on="Igraph" class="XYGraph (strict)"("YScale.Minimum"=w583) -> ()  [unwired: 2 in, 2 out]
            n318 = global read "QC_MeasurementSetup.vi" "IV Measurement Parameters"() -> (w582:T8)
            n319 = Unbundle By Name(w582) -> ("Number Of Steps"=w579:u32)
            n320 = local read "hold steps"() -> (w578:i32)
            n321 = Add(x=w579, y=w578) -> (x+y=w577:u32)
            n322 = call "IVData.vi"("Action"=w580, "Array No."=u32 1 ("Action")) -> ("Array OUT"=w589:dbl[])  [unwired: 3 in, 1 out]
            n323 = Array Subset(array=w589, index=0, length=w577) -> (w586:dbl[])
            n324 = Absolute Value(x=w586) -> (abs(x)=w585:dbl[])
            n325 = case shown="\"microAmps\"" w587 {
              tunnel: [w592 w593 w597] -> w591
              tunnel: w585 -> [w592 w595 w598]
              frame .."nanoAmps" {
              }
              frame "microAmps" {
                n326 = Divide(x=w595, y=1000.0) -> (x/y=w593:dbl[])
              }
              frame "milliAmps".. {
                n327 = Divide(x=w598, y=1000000.0) -> (x/y=w597:dbl[])
              }
            }
            n328 = call "IVData.vi"("Action"=w580, "Array No."=u32 0 ("Action")) -> ("Array OUT"=w576:dbl[])  [unwired: 3 in, 1 out]
            n329 = Absolute Value(x=w576) -> (abs(x)=w575:dbl[])
            n330 = Bundle(w575, w591) -> (w588:cluster{dbl[], dbl[]})  [unwired: 1 in]
            n331 = local write "Igraph"(w588) -> ()
          }
        }
        n332 = Not Or(1:"quit (no save)", 2:"Quit & Save") -> (0:w569:bool)
      }
      n333 = global read "QC_MeasurementSetup.vi" "IV Measurement Parameters"() -> (w522:T8)
      n334 = Unbundle By Name(w522) -> ("Temperature Readout"=w521:enum16{"Read Arduino", "Enter manually"}, "Arduino"=w515:refnum<class "ArduinoControl.lvclass">)
      n335 = case shown="\"Read Arduino\"" w521 {
        tunnel: w515 -> [_ w565]
        frame "Enter manually", Default {
        }
        frame "Read Arduino" {
          n336 = call "ArduinoClose.vi"("ArduinoControl in"=w565) -> ()  [unwired: 9 in, 2 out]
        }
      }
      n337 = case shown="True" w525 {
        tunnel: [FALSE w609] -> w527
        frame False {
        }
        frame True {
          n338 = Two Button Dialog(message="Are you sure you don't want to save the data?", 1:"Quit" ("F button name (\"Cancel\")"), 2:"Save data" ("T button name (\"OK\")")) -> (T button?=w609:bool)
        }
      }
      n339 = Or(x=w526, y=w527) -> (x .or. y?=w520:bool)
      n340 = flat-sequence {
        tunnel: w520 -> [w529]
        tunnel: [w529] -> w516
        tunnel: [TRUE] -> w514
        frame #0 {
          n341 = global read "QC_MeasurementSetup.vi" "IV Measurement Parameters"() -> (w539:T8)
          n342 = Unbundle By Name(w539) -> ("V_breakdown Limit [V]"=w533:dbl, "Number Of Steps"=w534:u32)
          n343 = call "ScanFeedback.vi"("measurement type"=T5."IV") -> ("V breakdown"=w531:dbl)  [unwired: 4 in, 4 out]
          n344 = case shown="True" w529 {
            tunnel: ["" w564] -> w540
            tunnel: [_ w547] -> w538
            tunnel: w534 -> [_ w545]
            frame False {
            }
            frame True {
              w559 = T3."Read Array" ("Action")
              n345 = local write "STATUS 1"("Saving Data ...") -> ()
              n346 = call "IVData.vi"("Action"=w559, "Array No."=u32 0 ("Action")) -> ("Array OUT"=w554:dbl[])  [unwired: 3 in, 1 out]
              n347 = call "IVData.vi"("Action"=w559, "Array No."=u32 1 ("Action")) -> ("Array OUT"=w553:dbl[])  [unwired: 3 in, 1 out]
              n348 = local read "hold steps"() -> (w544:i32)
              n349 = Build Array(w554, w553) -> (w552:dbl[][])
              n350 = call "IVData.vi"("Action"=w559, "Array No."=u32 3 ("Action")) -> ("Array OUT"=w561:dbl[])  [unwired: 3 in, 1 out]
              n351 = call "IVData.vi"("Action"=w559, "Array No."=u32 2 ("Action")) -> ("Array OUT"=w560:dbl[])  [unwired: 3 in, 1 out]
              n352 = Add(x=w545, y=w544) -> (x+y=w543:u32)
              n353 = call <vilib>:"Std Deviation and Variance.vi"("X"=w561) -> ("mean"=w548:dbl)  [unwired: 1 in, 2 out]
              n354 = call <vilib>:"Std Deviation and Variance.vi"("X"=w560) -> ("mean"=w549:dbl)  [unwired: 1 in, 2 out]
              n355 = Transpose 2D Array(2D array=w552) -> (transposed array=w551:dbl[][])
              n356 = call "SaveDataFile.vi"("Data Array"=w551, "Temperature"=w549, "Humidity"=w548, "no. of arrays"=2, "Actual array lengths"=w543, "Array Titles"="Voltage[V] Current[nA]", "Strip Segment"="", "Arrays format"="%010.2f") -> ("Path + Filename OUT"=w564:string, "Error Out"=w547:errorcluster)  [unwired: 4 in, 2 out]
            }
          }
          n357 = Absolute Value(x=w531) -> (abs(x)=w530:dbl)
          n358 = Absolute Value(x=w533) -> (abs(x)=w532:dbl)
          n359 = Greater Or Equal?(x=w530, y=w532) -> (x >= y?=w535:bool)
          n360 = call "WriteLogFile.vi"("Automatic warning"="", "Data File"=w540, "Error In"=w538, "DUT passed?"=w535, "Value TechSpec criteria"=w531, "Files saved?"=w529) -> ()  [unwired: 5 in, 1 out]
        }
      }
      n361 = Select(t="Run finished.\nData saved." ("STATUS 1"), s=w516, f="Run finished.\nData not saved." ("STATUS 1")) -> (s? t:f=w519:string)
      n362 = local write "STATUS 1"(w519) -> ()
      "Done!" <- w514
    }
  }
